vi "sub_getRN16.vi"(4 "threshold":dbl=0.004, 5 "low":dbl=0.175, 6 "avg factor":dbl=0.8, 8 "high":dbl=0.215, 9 "x factor":dbl=0.2, 10 "Raw Signal":dynamicdata(waveform)) -> (1 "Digitized Sign":dynamicdata(waveform), 2 "Moving Avg":dynamicdata(waveform), 3 "Bits":i16[](array[numeric]))   [LabVIEW 2015]
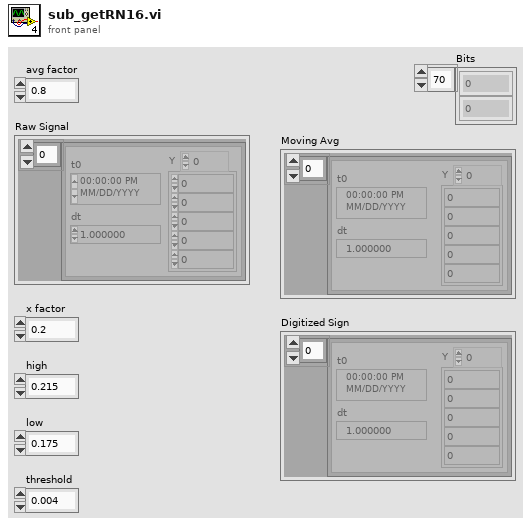
[diagram p1: front panel]
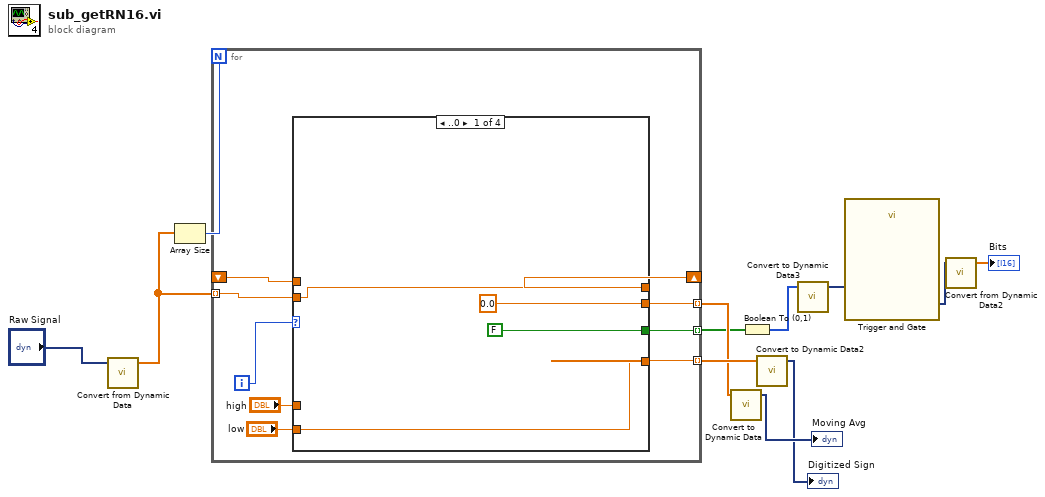
[diagram p0: block diagram]
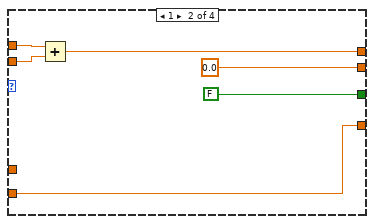
[diagram p2: hidden frame]
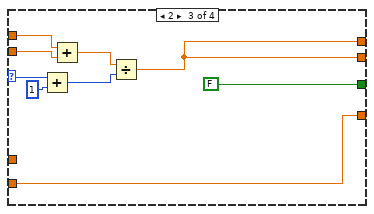
[diagram p3: hidden frame]
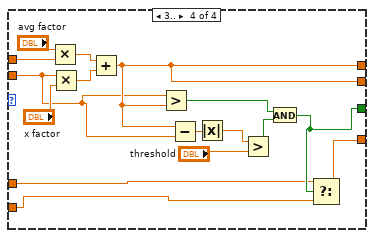
[diagram p4: hidden frame]
diagram:
  n1 = call "Convert from Dynamic Data"("Dynamic Data Type"="Raw Signal") -> ("Array"=w8:dbl[])  [unwired: 3 in]
  n2 = Array Size(array=w8) -> (size(s)=w7:i32)
  n3 = for {
    N: w7 -> [_]
    tunnel: w8 -> [w20] mode=indexing
    tunnel: [w19] -> w9 mode=indexing
    shift-right: [w17] -> _
    shift-left: _ -> [w18]
    tunnel: [w16] -> w4 mode=indexing
    tunnel: [w15] -> w12 mode=indexing
    i -> [w21]
    n4 = case shown="..0" w21 {
      selector: w21 -> [_ _ w37 _]
      tunnel: w20 -> [w24 w30 w36 w46]
      tunnel: [0.0 0.0 w34 w47] -> w19
      tunnel: w18 -> [_ w31 w35 w56]
      tunnel: [w24 w28 w34 w47] -> w17
      tunnel: [FALSE FALSE FALSE w43] -> w16
      tunnel: [w22 w26 w32 w51] -> w15
      tunnel: "high" -> [_ _ _ w42]
      tunnel: "low" -> [w22 w26 w32 w41]
      frame ..0 {
      }
      frame 1 {
        n5 = Add(x=w31, y=w30) -> (x+y=w28:dbl)
      }
      frame 2 {
        n6 = Add(x=w37, y=1) -> (x+y=w38:i32)
        n7 = Add(x=w35, y=w36) -> (x+y=w39:dbl)
        n8 = Divide(x=w39, y=w38) -> (x/y=w34:dbl)
      }
      frame 3.. {
        n9 = Multiply(x="avg factor", y=w56) -> (x*y=w53:dbl)
        n10 = Multiply(x=w46, y="x factor") -> (x*y=w52:dbl)
        n11 = Add(x=w53, y=w52) -> (x+y=w47:dbl)
        n12 = Greater?(x=w46, y=w47) -> (0:w44:bool)
        n13 = Subtract(x=w47, y=w46) -> (x-y=w50:dbl)
        n14 = Absolute Value(x=w50) -> (abs(x)=w49:dbl)
        n15 = Greater?(x=w49, y="threshold") -> (0:w45:bool)
        n16 = And(x=w44, y=w45) -> (x .and. y?=w43:bool)
        n17 = Select(t=w42, s=w43, f=w41) -> (s? t:f=w51:dbl)
      }
    }
  }
  n18 = call "Convert to Dynamic Data"("Array"=w9) -> ("Dynamic Data Type"=→"Moving Avg":dynamicdata)  [unwired: 3 in]
  n19 = Boolean To (0,1)(Boolean=w4) -> (0, 1=w6:i16[])
  n20 = call "Convert to Dynamic Data2"("Array"=w12) -> ("Dynamic Data Type"=→"Digitized Sign":dynamicdata)  [unwired: 3 in]
  n21 = call "Convert to Dynamic Data3"("Array"=w6) -> ("Dynamic Data Type"=w5:dynamicdata)  [unwired: 3 in]
  n22 = call "Trigger and Gate"("Signals"=w5) -> ("Triggered Signals"=w1:dynamicdata)  [unwired: 7 in, 3 out]
  n23 = call "Convert from Dynamic Data2"("Dynamic Data Type"=w1) -> ("Array"=→"Bits":dbl[])  [unwired: 3 in]
